vi "VIDescriptionEditor.vi"() -> ()   [LabVIEW 2021]
panel:
  in  "Refresh":bool
  in  "VI Search":string
  in  "UpdateAll":bool
  in  "Tree":string(tree)
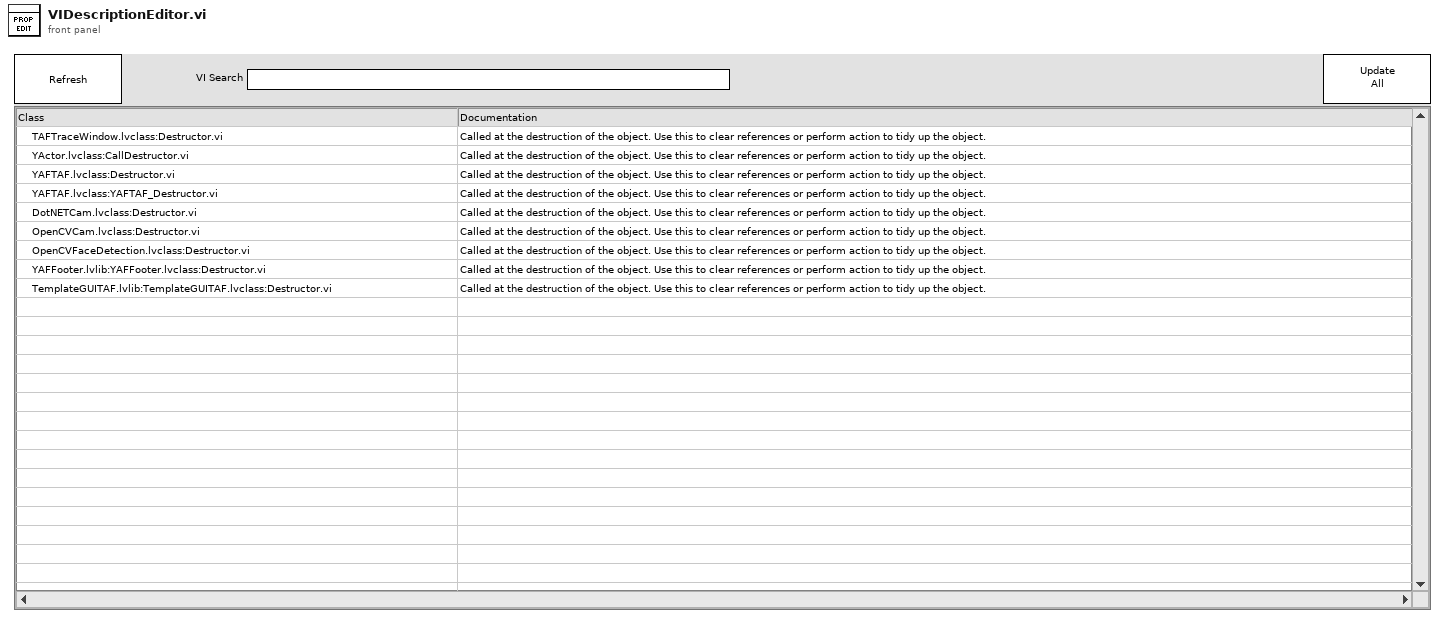
[diagram p1: front panel]
types:
  T1 = cluster{"Left Cell String":string, "Child Text":string[], "Child Tag":string, "Item Indent":i32, "Child Only?":bool, "Glyph Index":i32}
  T2 = cluster{"Project.ActiveProject":refnum<vi>, "My Computer":refnum<vi>, "All Descendents":refnum<vi>[], refnum<vi>[], refnum<vi>[]}
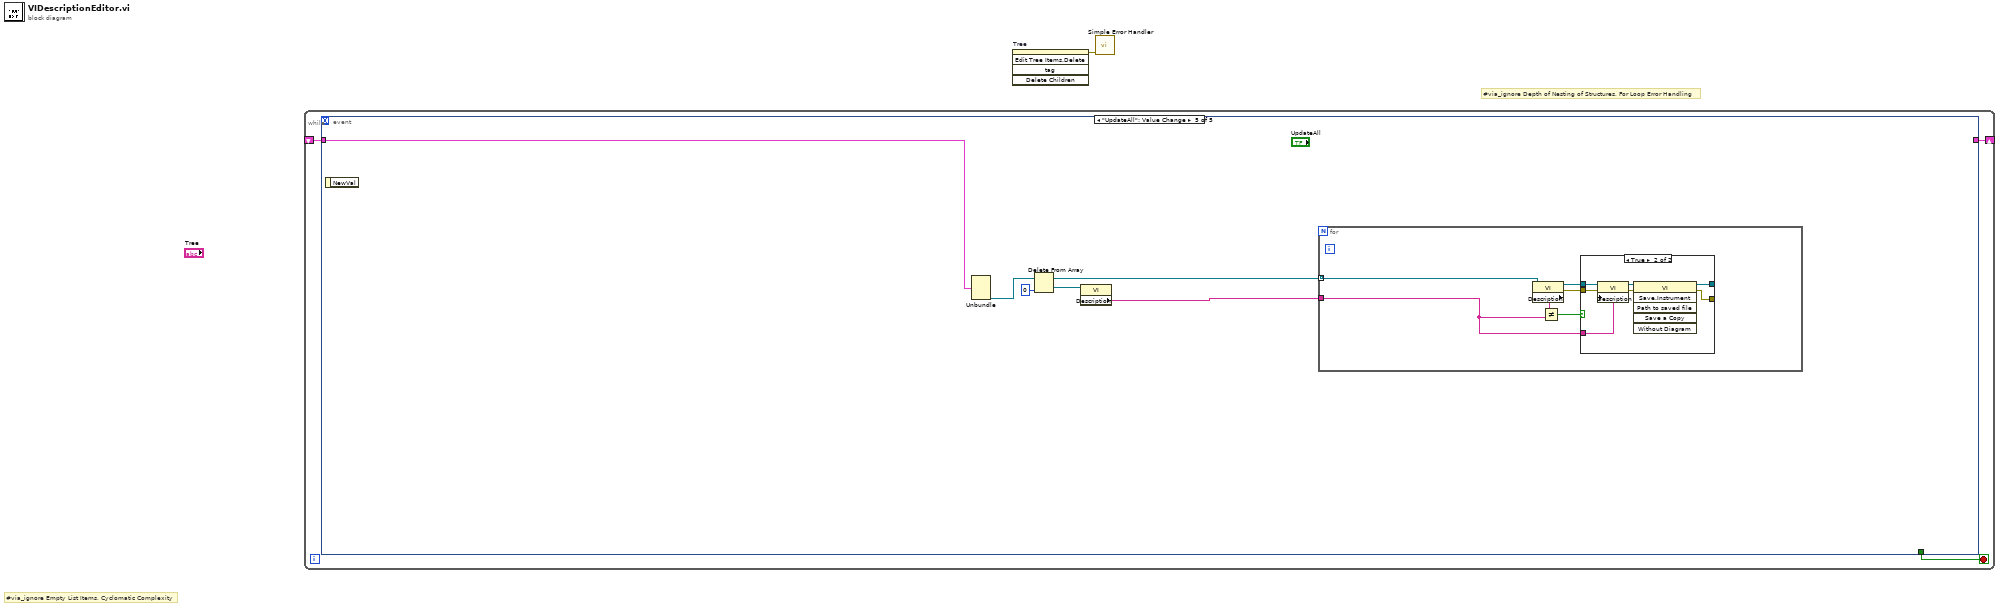
[diagram p0: block diagram]
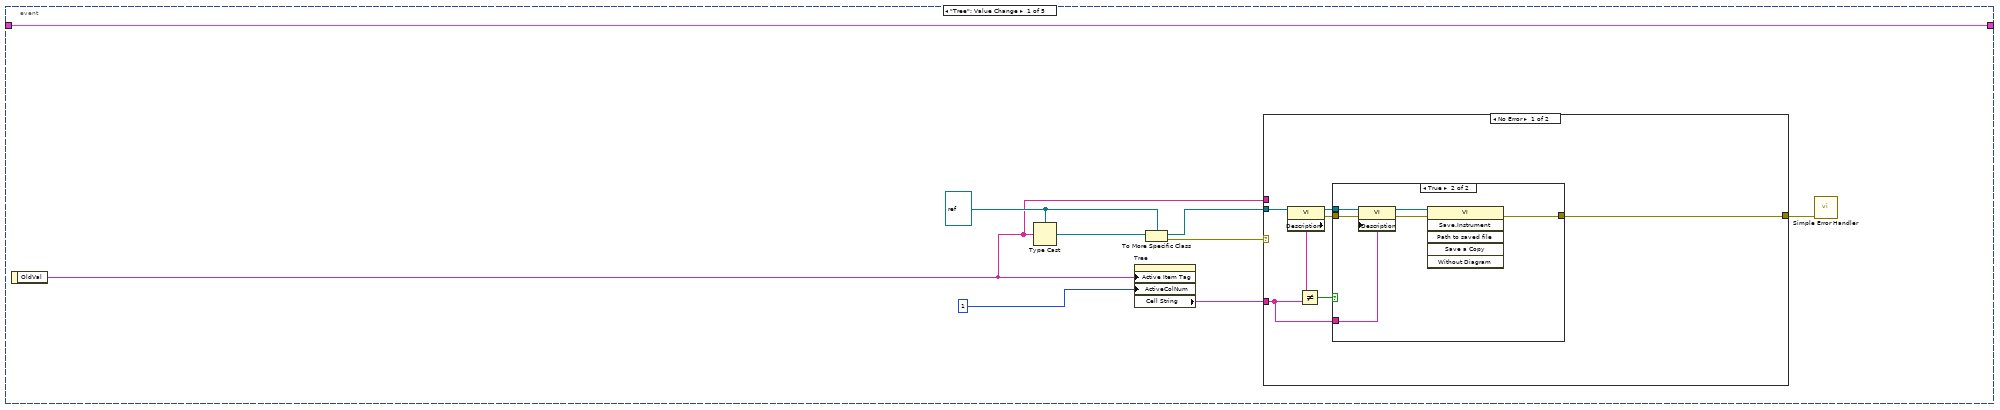
[diagram p2: hidden frame]
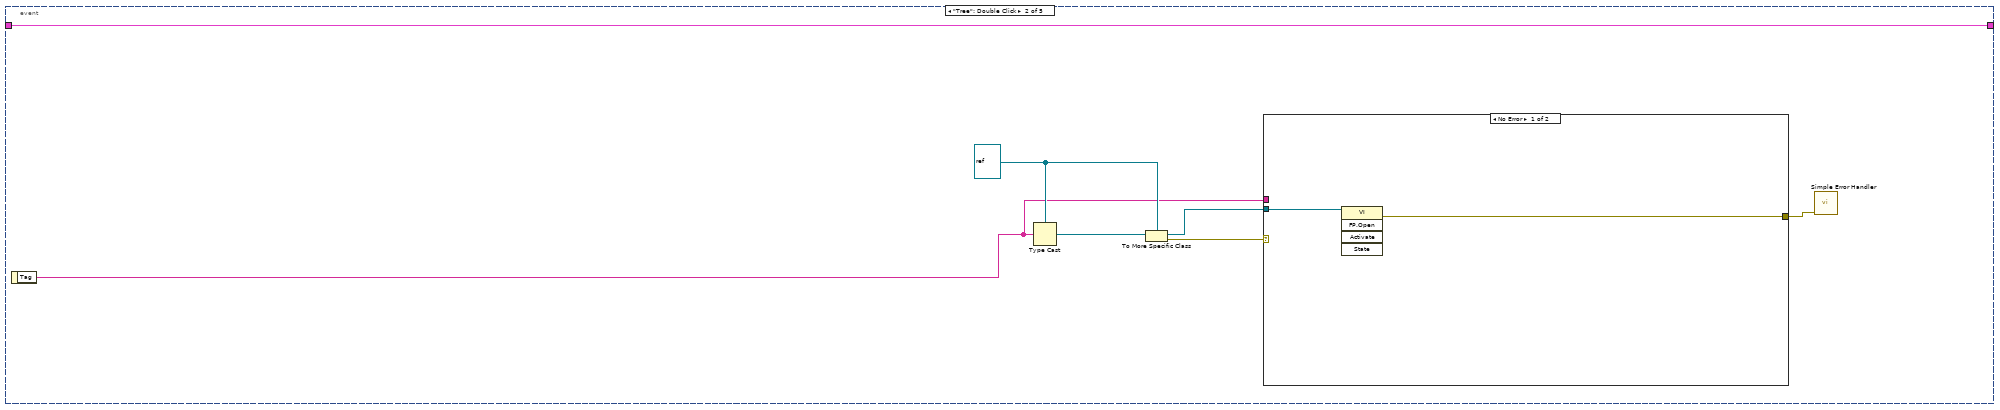
[diagram p5: hidden frame]
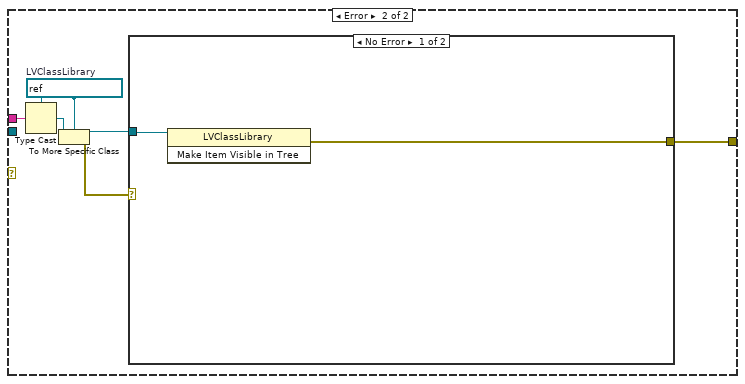
[diagram p6: hidden frame]
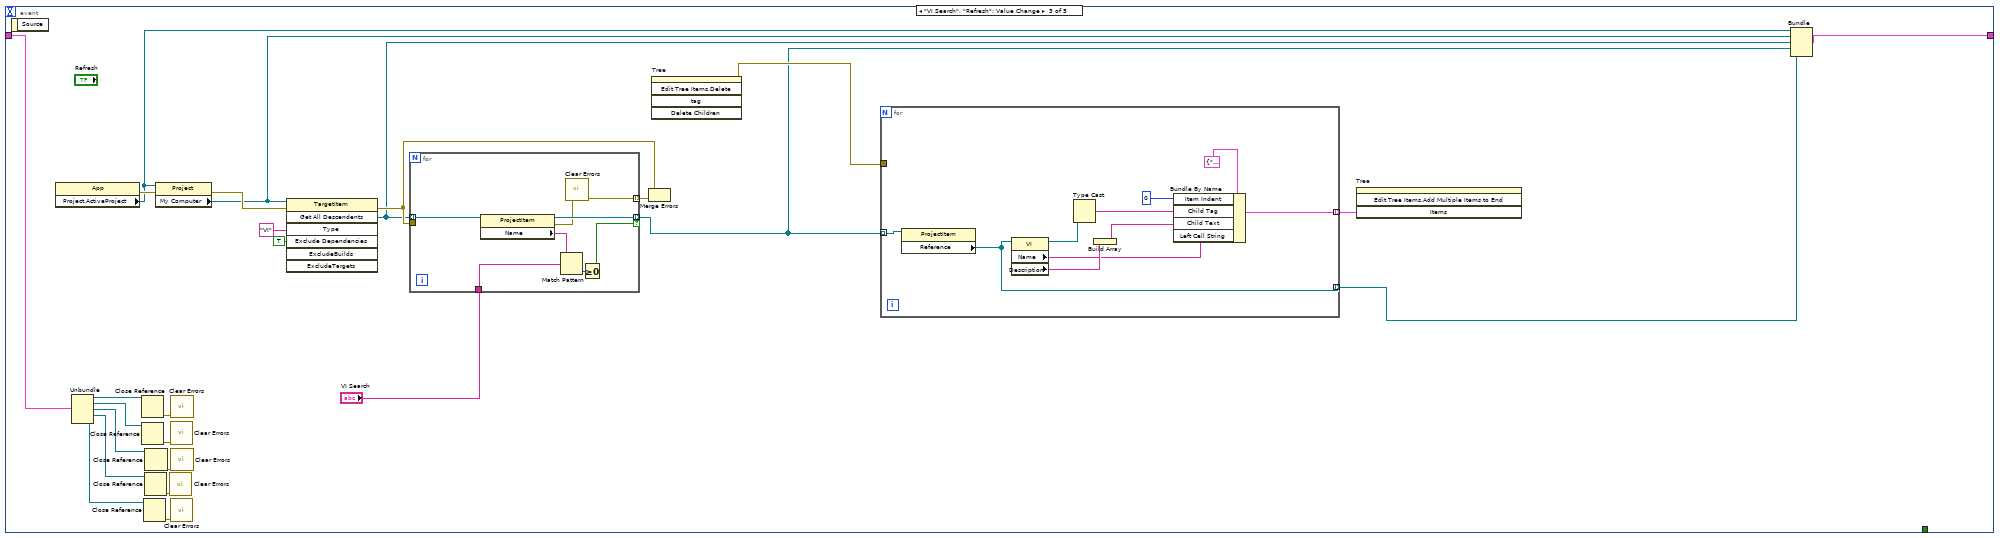
[diagram p8: hidden frame]
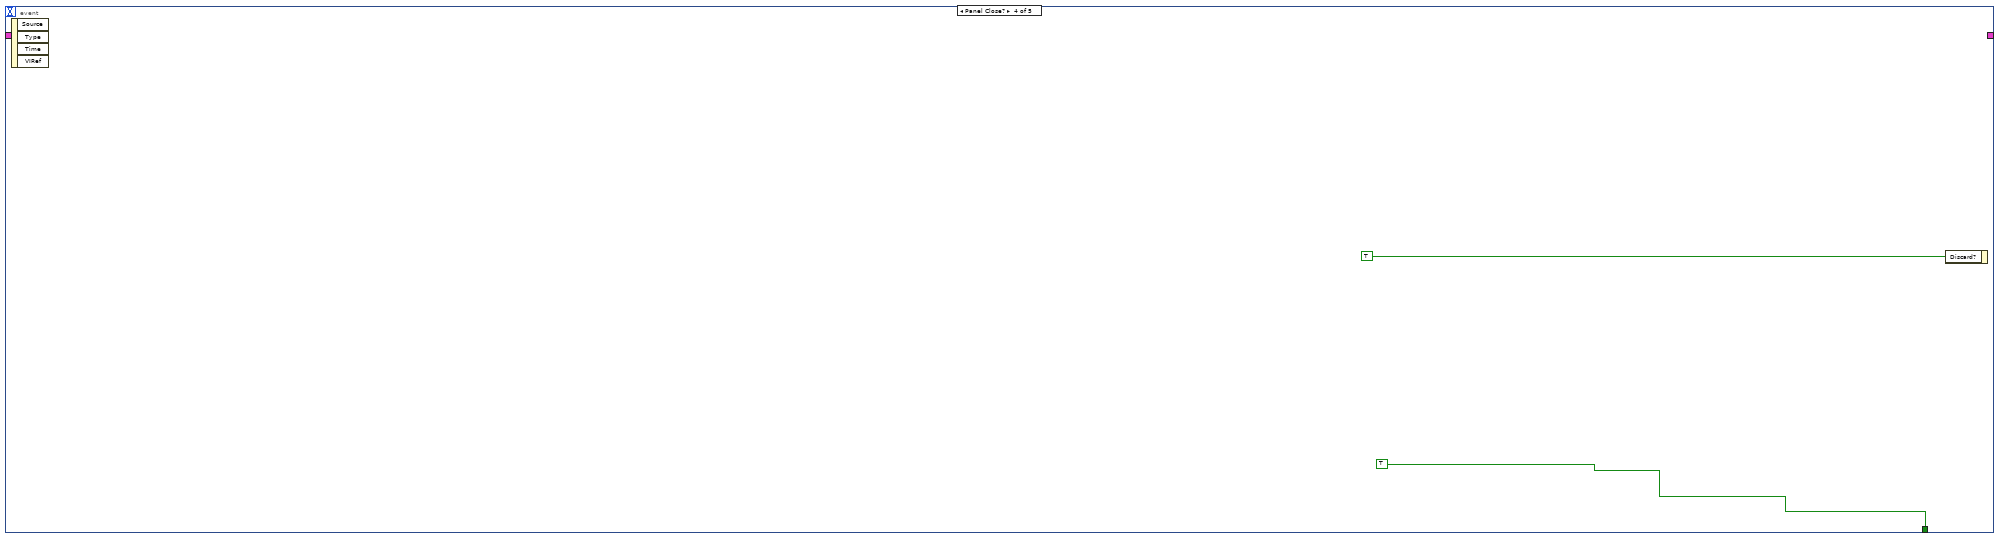
[diagram p9: hidden frame]
diagram:
  # "#via_ignore Depth of Nesting of Structures, For Loop Error Handling"
  # "#via_ignore Empty List Items, Cyclomatic Complexity"
  n1 = while {
    shift-right: [w4] -> _
    shift-left: _ -> [w3]
    stop <- w2 stop-if-true
    n2 = event shown="[4] \"UpdateAll\": Value Change" {
      selector: _ -> [_ _ _ _ _]
      dyn-events: _ -> [_ _ _ _ _]
      timeout: _ -> [_ _ _ _ _]
      tunnel: [w8 w31 w60 _ _] -> w4
      tunnel: w3 -> [w8 w31 w59 _ w95]
      tunnel: [_ _ _ TRUE _] -> w2
      event "Tree": Value Change {
        w12 = refnum<vi> refnum ("reference out")
        n3 = event-data() -> ("OldVal"=w6:string)  [unwired: 1 in]
        n4 = Type Cast(type=w12, x=w6) -> (*(type *) &x=w7:refnum<vi>)
        n5 = property on="Tree" class="Tree (strict)"("Active Item Tag"=w6, "ActiveColNum"=1 ("Active Cell:Active Column Number")) -> ("Cell String"=w9:string)  [unwired: 2 in, 2 out]
        n6 = To More Specific Class(target class=w12, reference=w7) -> (specific class reference=w10:refnum<vi>, error out=w11:errorcluster)  [unwired: 1 in]
        n7 = case shown="No Error" w11 {
          tunnel: w10 -> [w20 _]
          tunnel: w9 -> [w16 _]
          tunnel: w6 -> [_ _]
          tunnel: [w14 _] -> w5
          frame No Error {
            n8 = property class="VI"(reference=w20) -> (reference out=w17:refnum<vi>, error out=w15:errorcluster, "Description"=w19:string)  [unwired: 1 in]
            n9 = Not Equal?(x=w19, y=w16) -> (x != y?=w18:bool)
            n10 = case shown="True" w18 {
              tunnel: w17 -> [_ w27]
              tunnel: w16 -> [_ w26]
              tunnel: w15 -> [w21 w23]
              tunnel: [w21 w22] -> w14
              frame False {
              }
              frame True {
                n11 = property class="VI"(reference=w27, error in=w23, "Description"=w26) -> (reference out=w25:refnum<vi>, error out=w24:errorcluster)
                n12 = invoke class="VI" method="Save.Instrument"(reference=w25, error in=w24) -> (error out=w22:errorcluster)  [unwired: 4 in, 5 out]
              }
            }
          }
          frame Error {
          }
        }
        n13 = call <vilib>:"Simple Error Handler.vi"("error in (no error)"=w5) -> ()  [unwired: 4 in, 5 out]
      }
      event "Tree": Double Click {
        w34 = refnum<vi> refnum ("reference out")
        n14 = event-data() -> ("Tag"=w29:string)  [unwired: 1 in]
        n15 = Type Cast(type=w34, x=w29) -> (*(type *) &x=w30:refnum<vi>)
        n16 = To More Specific Class(target class=w34, reference=w30) -> (specific class reference=w32:refnum<vi>, error out=w33:errorcluster)  [unwired: 1 in]
        n17 = case shown="No Error" w33 {
          tunnel: w32 -> [w36 _]
          tunnel: w29 -> [_ w40]
          tunnel: [w35 w37] -> w28
          frame No Error {
            n18 = invoke class="VI" method="FP.Open"(reference=w36) -> (error out=w35:errorcluster)  [unwired: 4 in, 4 out]
          }
          frame Error {
            w38 = refnum<vi> refnum  # LVClassLibrary
            n19 = Type Cast(type=w38, x=w40) -> (*(type *) &x=w39:refnum<vi>)
            n20 = To More Specific Class(target class=w38, reference=w39) -> (specific class reference=w42:refnum<vi>, error out=w41:errorcluster)  [unwired: 1 in]
            n21 = case shown="No Error" w41 {
              tunnel: w42 -> [w44 _]
              tunnel: [w43 _] -> w37
              frame No Error {
                n22 = invoke class="LVClassLibrary" method="Make Item Visible in Tree"(reference=w44) -> (error out=w43:errorcluster)  [unwired: 2 in, 2 out]
              }
              frame Error {
              }
            }
          }
        }
        n23 = call <vilib>:"Simple Error Handler.vi"("error in (no error)"=w28) -> ()  [unwired: 4 in, 5 out]
      }
      event "VI Search", "Refresh": Value Change {
        w64 = TRUE ("ExcludeDependencies")
        n24 = event-data() -> ()  [unwired: 1 in, 1 out]
        n25 = property class="App"() -> (error out=w67:errorcluster, "Project.ActiveProject"=w63:refnum<vi>)  [unwired: 2 in, 1 out]
        n26 = Unbundle(w59) -> ("Project.ActiveProject"=w58:refnum<vi>, "My Computer"=w57:refnum<vi>, "All Descendents"=w56:refnum<vi>[], w55:refnum<vi>[], w48:refnum<vi>[])
        n27 = Close Reference(reference=w58) -> (error out=w54:errorcluster)  [unwired: 1 in]
        n28 = Close Reference(reference=w57) -> (error out=w53:errorcluster)  [unwired: 1 in]
        n29 = Close Reference(reference=w48) -> (error out=w50:errorcluster)  [unwired: 1 in]
        n30 = Close Reference(reference=w55) -> (error out=w51:errorcluster)  [unwired: 1 in]
        n31 = Close Reference(reference=w56) -> (error out=w52:errorcluster)  [unwired: 1 in]
        n32 = property class="Project"(reference=w63, error in=w67) -> (error out=w68:errorcluster, "My Computer"=w62:refnum<vi>)  [unwired: 1 out]
        n33 = call <vilib>:"Clear Errors.vi"("error in (no error)"=w51) -> ()  [unwired: 5 in, 2 out]
        n34 = call <vilib>:"Clear Errors.vi"("error in (no error)"=w53) -> ()  [unwired: 5 in, 2 out]
        n35 = call <vilib>:"Clear Errors.vi"("error in (no error)"=w50) -> ()  [unwired: 5 in, 2 out]
        n36 = call <vilib>:"Clear Errors.vi"("error in (no error)"=w54) -> ()  [unwired: 5 in, 2 out]
        n37 = call <vilib>:"Clear Errors.vi"("error in (no error)"=w52) -> ()  [unwired: 5 in, 2 out]
        n38 = invoke class="TargetItem" method="Get All Descendents"(reference=w62, error in=w68, "Type"="VI", "Exclude Dependencies"=w64, "ExcludeBuilds"=w64, "ExcludeTargets"=w64) -> (error out=w69:errorcluster, "All Descendents"=w61:refnum<vi>[])  [unwired: 1 in, 5 out]
        n39 = for {
          tunnel: w61 -> [w81] mode=indexing
          tunnel: [w87] -> w46 mode=indexing if=w85
          tunnel: w69 -> [_]
          tunnel: "VI Search" -> [w83]
          tunnel: [w82] -> w47 mode=indexing
          n40 = property class="ProjectItem"(reference=w81) -> (reference out=w87:refnum<vi>, error out=w84:errorcluster, "Name"=w88:string)  [unwired: 1 in]
          n41 = Match Pattern(string=w88, regular expression=w83) -> (offset past match=w86:i32)  [unwired: 1 in, 3 out]
          n42 = call <vilib>:"Clear Errors.vi"("error in (no error)"=w84) -> ("error out"=w82:errorcluster)  [unwired: 5 in, 1 out]
          n43 = Greater Or Equal To 0?(x=w86) -> (x >= 0?=w85:bool)
        }
        n44 = Merge Errors(w69, w47) -> ()  [unwired: 1 out]
        n45 = invoke on="Tree" class="Tree (strict)" method="Edit Tree Items.Delete"() -> (error out=w66:errorcluster)  [unwired: 5 in, 4 out]
        n46 = for {
          tunnel: w46 -> [w80] mode=indexing
          tunnel: w66 -> [_]
          tunnel: [w71] -> w49 mode=indexing
          tunnel: [w79] -> w45 mode=indexing
          n47 = property class="ProjectItem"(reference=w80) -> ("Reference"=w71:refnum<vi>)  [unwired: 1 in, 2 out]
          n48 = property class="VI"(reference=w71) -> (reference out=w72:refnum<vi>, "Name"=w74:string, "Description"=w76:string)  [unwired: 1 in, 1 out]
          n49 = Type Cast(x=w72) -> (*(type *) &x=w73:string)  [unwired: 1 in]
          n50 = Build Array(w76) -> (w75:string[])
          n51 = Bundle By Name(cluster=T1 {"Left Cell String"="", "Child Text"=[], "Child Tag"="", "Item Indent"=0, "Child Only?"=FALSE, "Glyph Index"=0} ("Item"), "Item Indent"=0, "Child Tag"=w73, "Child Text"=w75, "Left Cell String"=w74) -> (w79:T1)
        }
        n52 = invoke on="Tree" class="Tree (strict)" method="Edit Tree Items.Add Multiple Items to End"("Items"=w45) -> ()  [unwired: 3 in, 4 out]
        n53 = Bundle("Project.ActiveProject"=w63, "My Computer"=w62, "All Descendents"=w61, w46, w49) -> (w60:T2)  [unwired: 1 in]
      }
      event Panel Close? {
        n54 = event-data() -> ()  [unwired: 1 in, 4 out]
        n55 = event-data("Discard?"=TRUE) -> ()  [unwired: 1 in, 1 out]
      }
      event "UpdateAll": Value Change {
        n56 = event-data() -> ()  [unwired: 1 in, 1 out]
        n57 = Unbundle(w95) -> (w94:refnum<vi>[])  [unwired: 4 out]
        n58 = Delete From Array(array=w94, index=0) -> (deleted portion=w96:refnum<vi>, array with subset deleted=w93:refnum<vi>[])  [unwired: 1 in]
        n59 = property class="VI"(reference=w96) -> ("Description"=w92:string)  [unwired: 1 in, 2 out]
        n60 = for {
          tunnel: w93 -> [w102] mode=indexing
          tunnel: w92 -> [w97]
          n61 = property class="VI"(reference=w102) -> (reference out=w100:refnum<vi>, error out=w101:errorcluster, "Description"=w99:string)  [unwired: 1 in]
          n62 = Not Equal?(x=w99, y=w97) -> (x != y?=w98:bool)
          n63 = case shown="True" w98 {
            tunnel: [w104 w109] -> _
            tunnel: [w103 w108] -> _
            tunnel: w101 -> [w103 w107]
            tunnel: w100 -> [w104 w106]
            tunnel: w97 -> [_ w105]
            frame False {
            }
            frame True {
              n64 = property class="VI"(reference=w106, error in=w107, "Description"=w105) -> (reference out=w111:refnum<vi>, error out=w110:errorcluster)
              n65 = invoke class="VI" method="Save.Instrument"(reference=w111, error in=w110) -> (reference out=w109:refnum<vi>, error out=w108:errorcluster)  [unwired: 4 in, 4 out]
            }
          }
        }
      }
    }
  }
  n66 = invoke on="Tree" class="Tree (strict)" method="Edit Tree Items.Delete"() -> (error out=w1:errorcluster)  [unwired: 5 in, 4 out]
  n67 = call <vilib>:"Simple Error Handler.vi"("error in (no error)"=w1) -> ()  [unwired: 4 in, 5 out]
